vi "start map.vi"(7 "spect_depth":u16, 8 "error in (no error)":errorcluster, 9 "points":u32, 10 "sp_time":u32, 11 "identifier":string) -> (0 "error out":errorcluster, 3 "function return":u32)   [LabVIEW 2015, in "XGL_DPP.lvlib"]
doc: "EXTERN DECLSPEC uint32_t CALL_CONV start_map(const char * identifier, const uint32_t sp_time, const uint32_t points, const uint16_t spect_depth);"
uses:
  XGL_DPP.lvlib
  XGL_DPP.dll
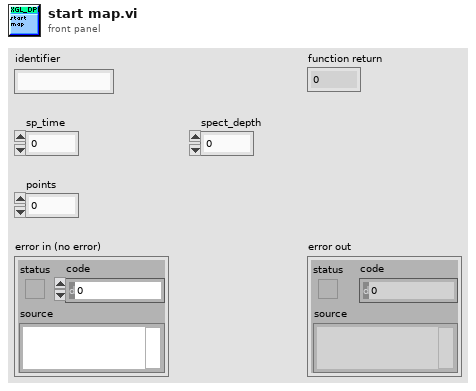
[diagram p1: front panel]
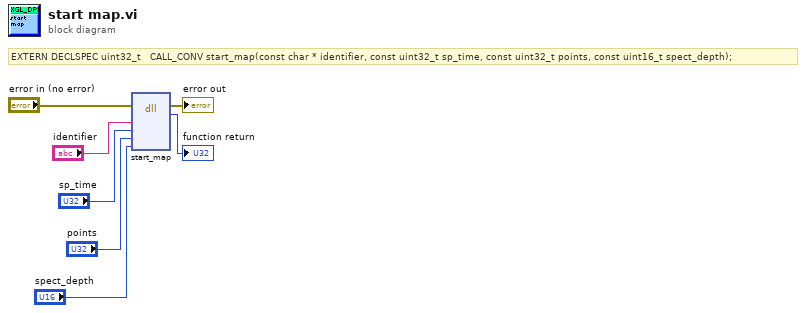
[diagram p0: block diagram]
diagram:
  # "EXTERN DECLSPEC uint32_t   CALL_CONV start_map(const char * identifier, const uint32_t sp_time, const uint32_t points, const uint16_t spect_depth);"
  n1 = dll-call lib="D:/Users/XRF/Desktop/Scanning Software_Demokritos_2015_v7/libs/Vis_2/XGL_DPP.*" fn="start_map"(error in="error in (no error)", "identifier"="identifier", "sp_time"="sp_time", "points"="points", "spect_depth"="spect_depth") -> (error out=→"error out":errorcluster, →"function return":u32)  [unwired: 6 in, 1 out]
